vi "Read_Out_FPGA.vi"(8 "Repetition Rate":bool, 10 "U8ReadFIFO":u8[](array[numeric]), 11 "U64ReadFIFO":u64[](array[numeric])) -> (2 "Trigger":bool[](array[boolean]), 3 "PMT Signal":u8[](array[numeric]))   [LabVIEW 2012]
panel:
  # "40MHz"
  # "80MHz"
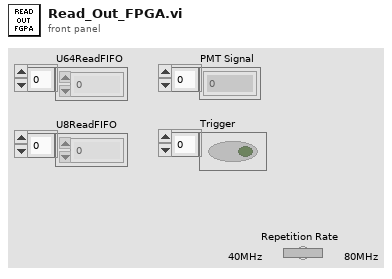
[diagram p1: front panel]
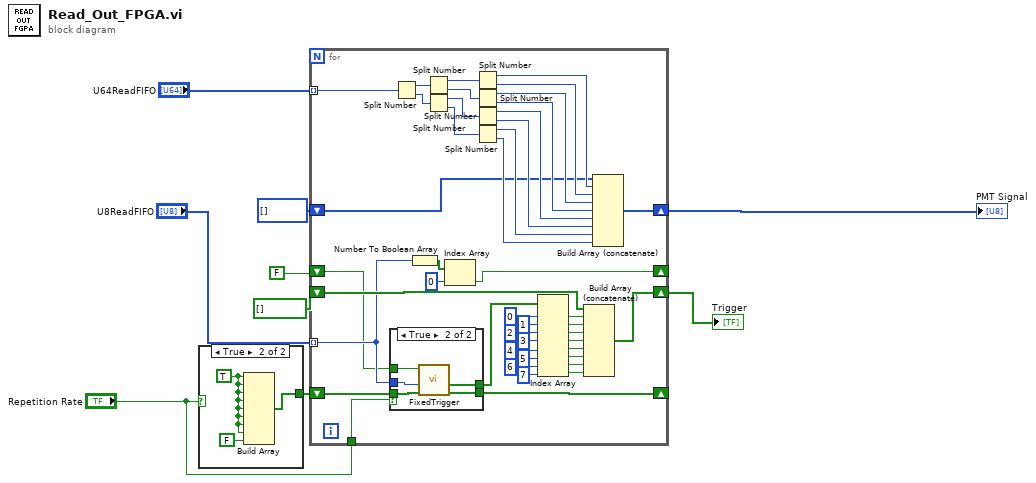
[diagram p0: block diagram]
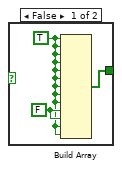
[diagram p2: hidden frame]
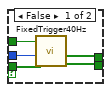
[diagram p3: hidden frame]
diagram:
  n1 = case shown="True" "Repetition Rate" {
    tunnel: [w12 w13] -> w3
    frame False {
      w11 = FALSE
      w10 = TRUE
      n2 = Build Array(w10, w10, w10, w10, w10, w10, w10, w10, w10, w11, w11, w10, w10) -> (w12:bool[])
    }
    frame True {
      w14 = TRUE
      n3 = Build Array(w14, w14, w14, w14, w14, w14, w14, w14, FALSE) -> (w13:bool[])
    }
  }
  n4 = for {
    tunnel: "U64ReadFIFO" -> [w59] mode=indexing
    shift-right: [w44] -> w9
    shift-left: u8[] [] -> [w43]
    tunnel: "U8ReadFIFO" -> [w21] mode=indexing
    shift-right: [w42] -> w8
    shift-left: bool[] [] -> [w41]
    shift-right: [w18] -> _
    shift-left: w3 -> [w19]
    shift-right: [w22] -> _
    shift-left: FALSE -> [w20]
    tunnel: "Repetition Rate" -> [w16]
    n5 = case shown="True" w16 {
      tunnel: w21 -> [w61 w69]
      tunnel: w20 -> [w62 w68]
      tunnel: w19 -> [w60 w67]
      tunnel: [w63 w66] -> w18
      tunnel: [w64 w65] -> w17
      frame False {
        n6 = call "FixedTrigger40Hz.vi"("array in"=w60, "IO Module\\Synchronous Trigger Input"=w61, "Last? Input"=w62) -> ("array out"=w63:bool[], "trigger out"=w64:bool[])  [unwired: 7 in]
      }
      frame True {
        n7 = call "FixedTrigger.vi"("array in"=w67, "IO Module\\Synchronous Trigger Input"=w69, "Last? Input"=w68) -> ("array out"=w66:bool[], "trigger out"=w65:bool[])  [unwired: 7 in]
      }
    }
    n8 = Split Number(x=w59) -> (hi(x)=w58:u32, lo(x)=w57:u32)
    n9 = Number To Boolean Array(number=w21) -> (Boolean array=w23:bool[])
    n10 = Split Number(x=w58) -> (hi(x)=w56:u16, lo(x)=w55:u16)
    n11 = Split Number(x=w57) -> (hi(x)=w54:u16, lo(x)=w53:u16)
    n12 = Index Array(array=w23, index=0) -> (element=w22:bool)
    n13 = Split Number(x=w56) -> (hi(x)=w52:u8, lo(x)=w51:u8)
    n14 = Split Number(x=w55) -> (hi(x)=w50:u8, lo(x)=w49:u8)
    n15 = Split Number(x=w54) -> (hi(x)=w48:u8, lo(x)=w47:u8)
    n16 = Split Number(x=w53) -> (hi(x)=w46:u8, lo(x)=w45:u8)
    n17 = Index Array(array=w17, index #1=0 ("index"), index #2=1 ("index"), index #3=2 ("index"), index #4=3 ("index"), index #5=4 ("index"), index #6=5 ("index"), index #7=6 ("index"), index #8=7 ("index")) -> (element #1=w32:bool, element #2=w31:bool, element #3=w30:bool, element #4=w29:bool, element #5=w28:bool, element #6=w27:bool, element #7=w26:bool, element #8=w25:bool)
    n18 = Build Array (concatenate)(w41, w32, w31, w30, w29, w28, w27, w26, w25) -> (w42:bool[])
    n19 = Build Array (concatenate)(w43, w52, w51, w50, w49, w48, w47, w46, w45) -> (w44:u8[])
  }
  "PMT Signal" <- w9
  "Trigger" <- w8
